vi "MoveJointsSubVI.vi"(0 "TCP Network Connection in":refnum<k5>, 1 "Theta1":dbl, 2 "Theta2":dbl, 3 "Theta3":dbl, 4 "Theta4":dbl, 5 "Theta5":dbl, 6 "Theta6":dbl, 7 "Send_command":bool) -> (20 "TCP Network Connection out":refnum<k5>, 23 "bytes written":i32, 27 "error out":errorcluster)   [LabVIEW 2020]
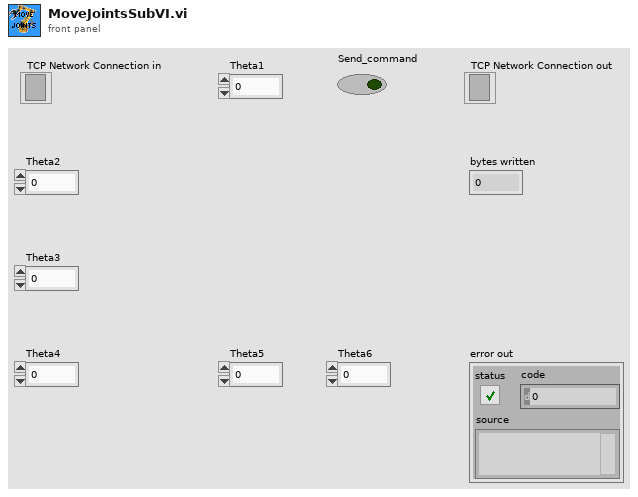
[diagram p1: front panel]
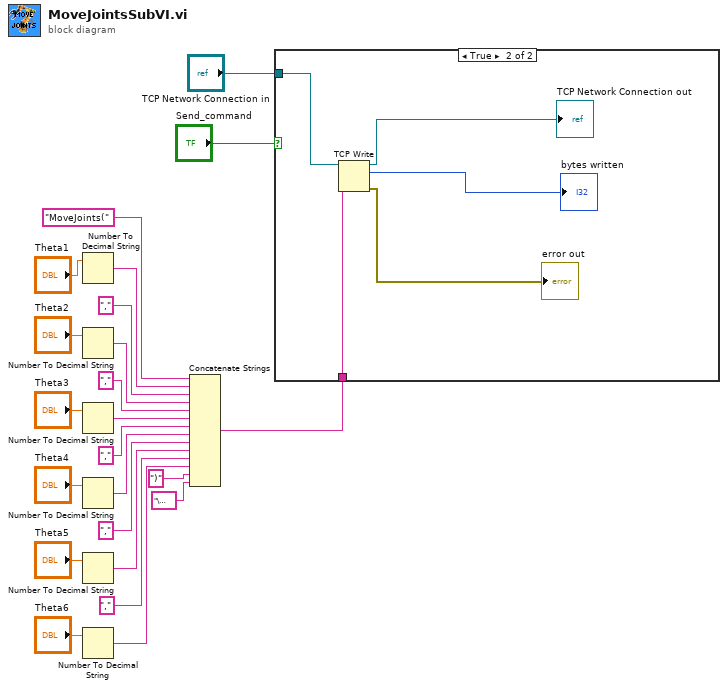
[diagram p0: block diagram]
diagram:
  n1 = Number To Decimal String(number="Theta1") -> (decimal integer string=w10:string)  [unwired: 1 in]
  n2 = Number To Decimal String(number="Theta2") -> (decimal integer string=w12:string)  [unwired: 1 in]
  n3 = Number To Decimal String(number="Theta3") -> (decimal integer string=w14:string)  [unwired: 1 in]
  n4 = Number To Decimal String(number="Theta4") -> (decimal integer string=w16:string)  [unwired: 1 in]
  n5 = Number To Decimal String(number="Theta5") -> (decimal integer string=w18:string)  [unwired: 1 in]
  n6 = Number To Decimal String(number="Theta6") -> (decimal integer string=w20:string)  [unwired: 1 in]
  n7 = Concatenate Strings("MoveJoints(", w10, ",", w12, ",", w14, ",", w16, ",", w18, ",", w20, ")", "\u0000") -> (w23:string)
  n8 = case shown="True" "Send_command" {
    tunnel: "TCP Network Connection in" -> [_ w28]
    tunnel: w23 -> [_ w27]
    frame False {
    }
    frame True {
      n9 = TCP Write(connection ID=w28, data in=w27) -> (connection ID out=→"TCP Network Connection out":refnum<k5>, bytes written=→"bytes written":i32, error out=→"error out":errorcluster)  [unwired: 2 in]
    }
  }
